vi "DSF.Engine.Interface.Plugin.Write.Error.vi"(8 "error in (no error)":errorcluster, 9 "timeout in ms (0)":i32, 10 "error":errorcluster, 11 "Plugin Interface in":refnum<class "DSF.Engine.Interface.Plugin.lvclass">) -> (0 "error out":errorcluster, 1 "empty?":bool, 3 "Plugin Interface out":refnum<class "DSF.Engine.Interface.Plugin.lvclass">)   [LabVIEW 2017, in "DSF.Engine.lvlib" / "DSF.Engine.Interface.Plugin.lvclass"]
uses:
  DSF.Engine.Interface.Plugin.lvclass
  C:/Git/DSF/Source/Engine/Classes/Interface/DSF.Engine.Interface.lvclass
  DSF.Engine.Interface.lvclass/DSF.Engine.Interface.ctl
  DSF.Engine.Interface.lvclass
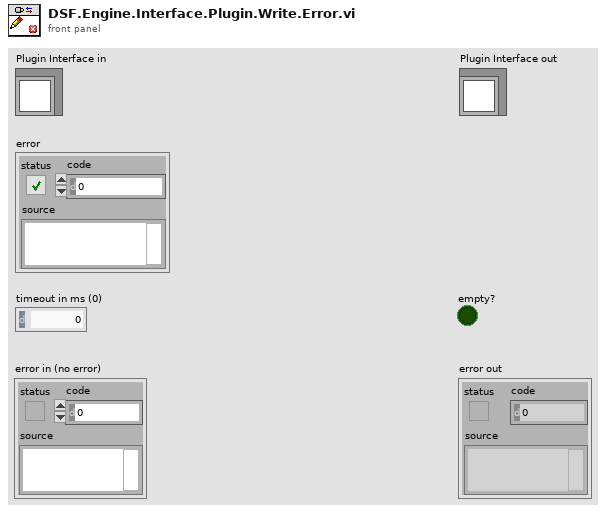
[diagram p1: front panel]
types:
  T1 = typedef "DSF.Engine.lvlib/DSF.Engine.Interface.lvclass/DSF.Engine.Interface.Error Queue.Ref.ctl" = refnum<queue>
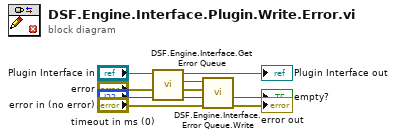
[diagram p0: block diagram]
diagram:
  n1 = call "DSF.Engine.Interface.Get Error Queue.vi"("Interface in"="Plugin Interface in") -> ("Error Queue"=w7:T1, "Interface out"=→"Plugin Interface out":refnum<class "DSF.Engine.Interface.Plugin.lvclass">)  [unwired: 9 in]
  n2 = call "DSF.Engine.Interface.Error Queue.Write.vi"("error in (no error)"="error in (no error)", "timeout in ms (0)"="timeout in ms (0)", "element"="error", "Error Queue in"=w7) -> ("error out"=→"error out":errorcluster, "timed out?"=→"empty?":bool)  [unwired: 5 in, 1 out]
